vi "gate_valve2.vi"(0 "Open Valve?":bool, 3 "physical channels":tag) -> ()   [LabVIEW 2014]
uses:
  <vilib>/DAQmx/create/channels.llb/DAQmx Create Channel (DO-Digital Output).vi
  <vilib>/DAQmx/write.llb/DAQmx Write (Digital Bool 1Line 1Point).vi
panel:
  in  "stop (F)":bool
  in  "timeout":dbl=10.0 format="%0.2f"
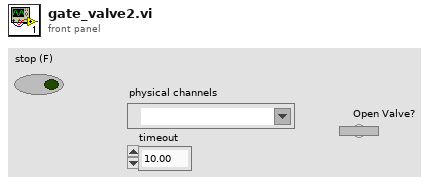
[diagram p1: front panel]
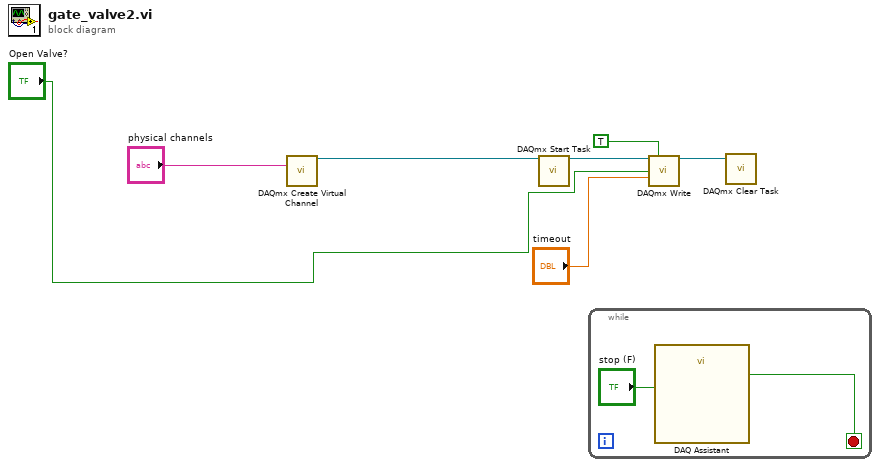
[diagram p0: block diagram]
diagram:
  n1 = call-poly <vilib>:"DAQmx Create Virtual Channel.vi"("lines"="physical channels") -> ("task out"=w1:refnum<k21>)  [unwired: 13 in, 1 out]
  n2 = call <vilib>:"DAQmx Start Task.vi"("task/channels in"=w1) -> ("task out"=w6:refnum<k21>)  [unwired: 13 in, 1 out]
  n3 = while {
    stop <- w8 stop-if-true
    n4 = call "DAQ Assistant"("stop (F)"="stop (F)") -> ("stopped"=w8:bool)  [unwired: 16 in, 2 out]
  }
  n5 = call-poly <vilib>:"DAQmx Write.vi"("task/channels in"=w6, "auto start"=TRUE, "data"="Open Valve?", "timeout"="timeout") -> ("task out"=w3:refnum<k21>)  [unwired: 9 in, 2 out]
  n6 = call <vilib>:"DAQmx Clear Task.vi"("task in"=w3) -> ()  [unwired: 14 in, 1 out]
